vi "Read Tab Selection.vi"(8 "error in (no error)":errorcluster, 11 "Settings in":refnum<class "Settings.lvclass">) -> (0 "error out":errorcluster, 2 "Tab Selection":T1(ring), 3 "Settings out":refnum<class "Settings.lvclass">)   [LabVIEW 2023, in "GUI.lvlib" / "Settings.lvlib" / "Settings.lvclass"]
uses:
  Settings.lvclass
  Settings.lvclass/Settings.ctl
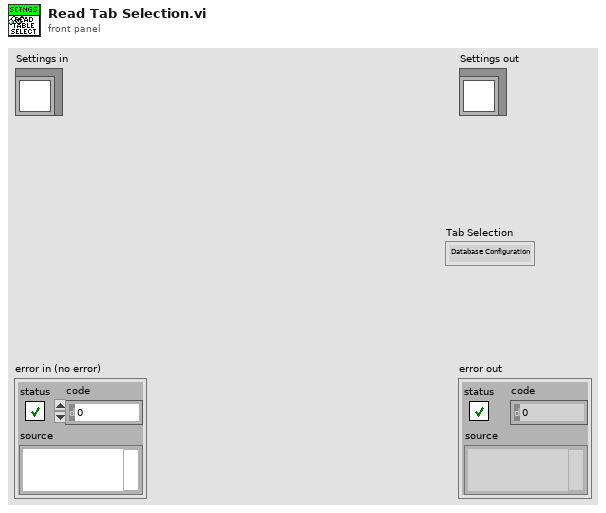
[diagram p1: front panel]
types:
  T1 = enum32{"Database Configuration", "DAQ Configuration"}
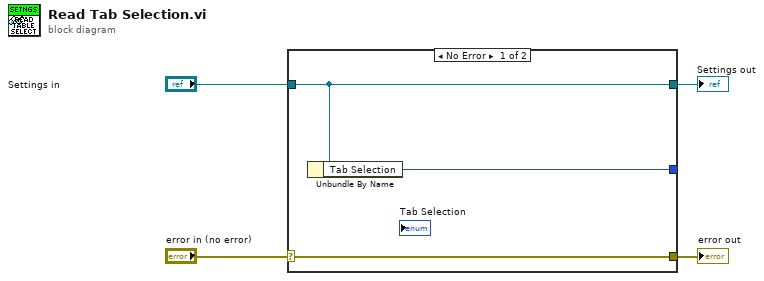
[diagram p0: block diagram]
diagram:
  n1 = case shown="No Error" "error in (no error)" {
    selector: "error in (no error)" -> [w7 w8]
    tunnel: [w7 w8] -> w3
    tunnel: [w6 w9] -> w1
    tunnel: "Settings in" -> [w6 w9]
    tunnel: [w5 _] -> _
    frame No Error {
      n2 = Unbundle By Name(w6) -> ("Tab Selection"=w5:T1)
    }
    frame Error {
    }
  }
  "error out" <- w3
  "Settings out" <- w1
